vi "Pick Best Candidates.vi"(7 "Markov Chain":T1, 10 "length":i32, 11 "Candidate Map":map{i32, string[][]}(c390)) -> (3 "Winners":cluster{"Class Name":string, "Count":i32}[](array[cluster]))   [LabVIEW 2024]
uses:
  Markov Chain.ctl
  <vilib>/Utility/miscctls.llb/LVMapReplaceAction.ctl
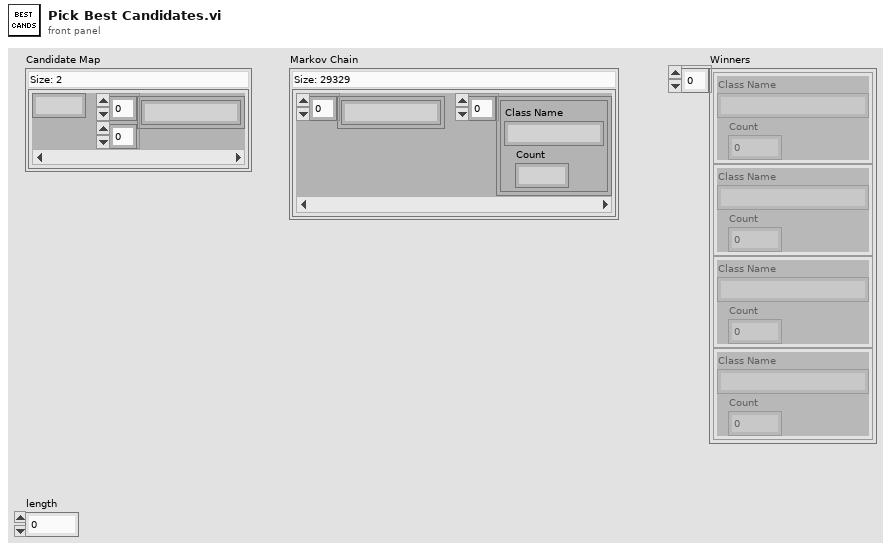
[diagram p1: front panel]
types:
  T1 = typedef "Markov Chain.ctl" = map{string[], cluster{"Class Name":string, "Count":i32}[]}
  T2 = typedef "LVMapReplaceAction.ctl" = enum32{"Modify Entry only if found", "Add or Modify Entry", "Delete Entry"}
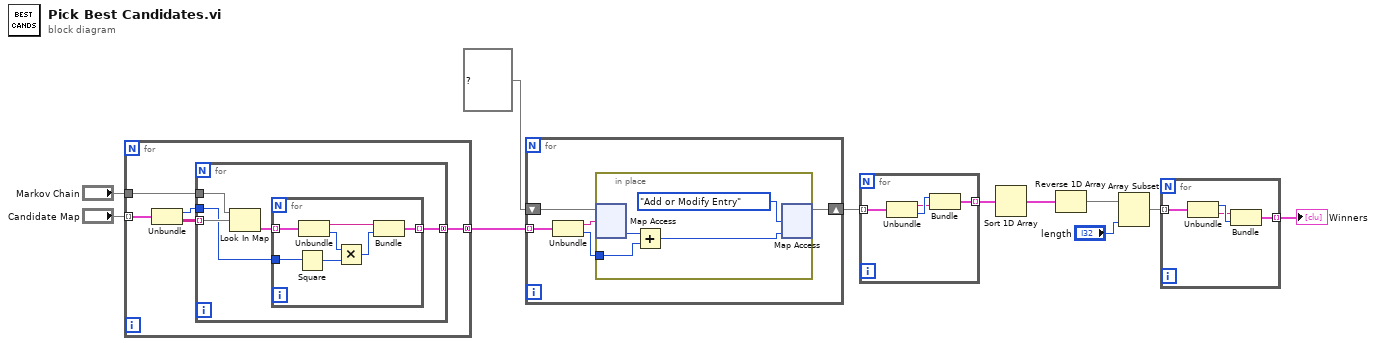
[diagram p0: block diagram]
diagram:
  n1 = for {
    tunnel: "Markov Chain" -> [w16]
    tunnel: [w15] -> w10 mode=concatenating
    tunnel: "Candidate Map" -> [w14] mode=indexing
    n2 = Unbundle(w14) -> ("Order"=w12:i32, "Candidates"=w13:string[][])
    n3 = for {
      tunnel: w16 -> [w20]
      tunnel: [w17] -> w15 mode=concatenating
      tunnel: w13 -> [w21] mode=indexing
      tunnel: w12 -> [w18]
      n4 = Look In Map(map=w20, key=w21) -> (value=w19:cluster{"Class Name":string, "Count":i32}[])  [unwired: 1 in, 1 out]
      n5 = for {
        tunnel: w19 -> [w28] mode=indexing
        tunnel: w18 -> [w26]
        tunnel: [w22] -> w17 mode=indexing
        n6 = Square(x=w26) -> (x^2=w24:i32)
        n7 = Unbundle(w28) -> ("Class Name"=w27:string, "Count"=w25:i32)
        n8 = Multiply(x=w25, y=w24) -> (x*y=w23:i32)
        n9 = Bundle("Class Name"=w27, w23) -> (w22:cluster{"Class Name":string, i32})  [unwired: 1 in]
      }
    }
  }
  n10 = for {
    tunnel: w10 -> [w33] mode=indexing
    shift-right: [w29] -> w8
    shift-left: map{string, i32} {} ("Map") -> [w30]
    n11 = Unbundle(w33) -> ("Class Name"=w32:string, w31:i32)
    n12 = in-place {
      in-place-border: w31 -> [w35]
      n13 = in-place-map #1(w30, w32) -> (w36:i32)  [unwired: 1 in, 1 out]
      n14 = Add(x=w36, y=w35) -> (x+y=w34:i32)
      n15 = in-place-map #1(w34, LVMapReplaceAction."Add or Modify Entry" ("action")) -> (w29:map{string, i32})  [unwired: 2 out]
    }
  }
  n16 = for {
    tunnel: w8 -> [w41] mode=indexing
    tunnel: [w38] -> w7 mode=indexing
    n17 = Unbundle(w41) -> (w39:string, w40:i32)
    n18 = Bundle(w40, w39) -> (w38:cluster{i32, string})  [unwired: 1 in]
  }
  n19 = Sort 1D Array(array=w7) -> (sorted array=w2:cluster{i32, string}[])
  n20 = Reverse 1D Array(array=w2) -> (reversed array=w1:cluster{i32, string}[])
  n21 = Array Subset(array=w1, length="length") -> (w5:cluster{i32, string}[])  [unwired: 1 in]
  n22 = for {
    tunnel: w5 -> [w45] mode=indexing
    tunnel: [w42] -> w4 mode=indexing
    n23 = Unbundle(w45) -> (w44:i32, w43:string)
    n24 = Bundle(w43, w44) -> (w42:cluster{string, i32})  [unwired: 1 in]
  }
  "Winners" <- w4
